vi "meta_findFirstBlock.vi"(8 "error in":errorcluster, 10 "block type":T2, 11 "meta file in":T3) -> (0 "error out":errorcluster, 1 "index":i32, 2 "block out":T1={"Version"=14, "Type"=enum."File", "Length"=0, "Data"=""}, 3 "meta file out":T3)   [LabVIEW 2017, in "NI_ExcelFile.lvlib"]
uses:
  <vilib>/express/express shared/NI_ExcelFile/NI_ExcelFile.lvlib
  <vilib>/express/express shared/NI_ExcelFile/Ctrls/meta_BlockType.ctl
  <vilib>/express/express shared/NI_ExcelFile/Ctrls/meta_file.ctl
  <vilib>/express/express shared/NI_ExcelFile/Ctrls/meta_Block.ctl
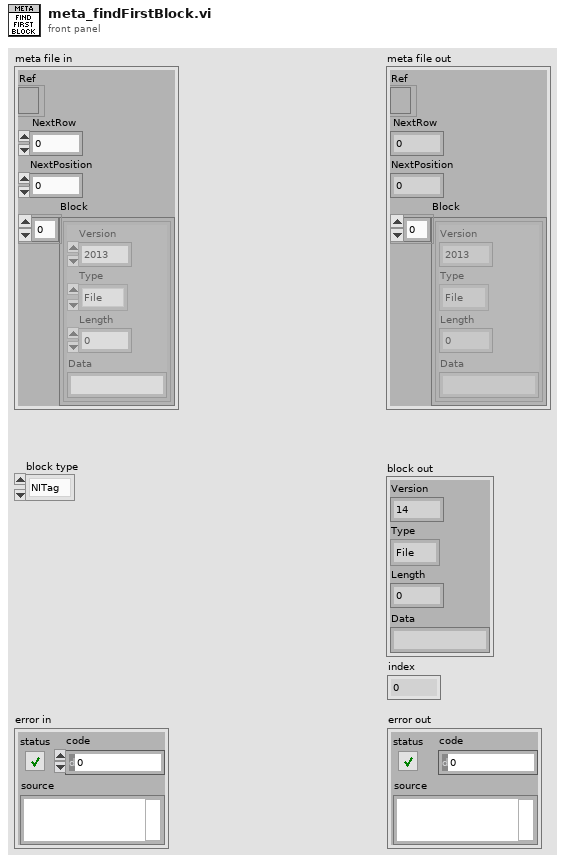
[diagram p1: front panel]
types:
  T1 = typedef "NI_ExcelFile.lvlib/meta_Block.ctl" = cluster{"Version":u16, "Type":T2, "Length":i32, "Data":string}
  T2 = typedef "NI_ExcelFile.lvlib/meta_BlockType.ctl" = enum16{"NITag", "File", "Column"}
  T3 = typedef "NI_ExcelFile.lvlib/meta_file.ctl" = cluster{"Ref":refnum<file>, "NextRow":i32, "NextPosition":i64, "Block":T1[]}
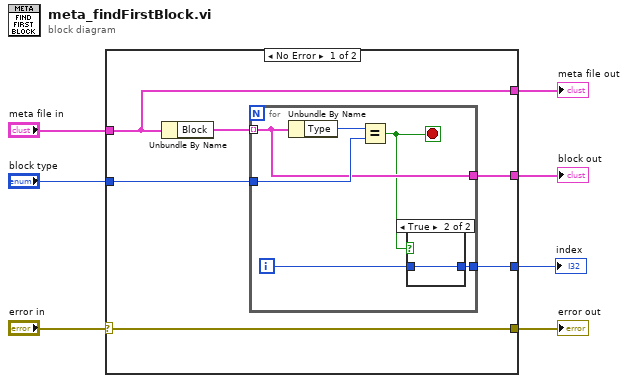
[diagram p0: block diagram]
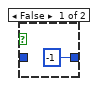
[diagram p2: hidden frame]
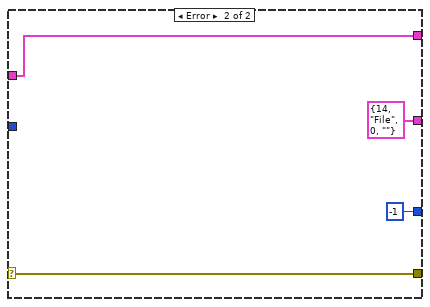
[diagram p3: hidden frame]
diagram:
  n1 = case shown="No Error" "error in" {
    selector: "error in" -> [w11 w25]
    tunnel: [w11 w25] -> w6
    tunnel: "meta file in" -> [w9 w24]
    tunnel: "block type" -> [w12 _]
    tunnel: [w10 T1 {"Version"=14, "Type"=enum."File", "Length"=0, "Data"=""} ("Block")] -> w3
    tunnel: [w9 w24] -> w2
    tunnel: [w8 -1] -> w1
    frame No Error {
      n2 = Unbundle By Name(w9) -> ("Block"=w13:T1[])
      n3 = for {
        tunnel: w13 -> [w17] mode=indexing
        tunnel: w12 -> [w18]
        tunnel: [w17] -> w10
        tunnel: [w15] -> w8
        i -> [w14]
        stop <- w16 stop-if-true
        n4 = Unbundle By Name(w17) -> ("Type"=w19:T2)
        n5 = Equal?(x=w19, y=w18) -> (x = y?=w16:bool)
        n6 = case shown="True" w16 {
          tunnel: [-1 w21] -> w15
          tunnel: w14 -> [_ w21]
          frame False {
          }
          frame True {
          }
        }
      }
    }
    frame Error {
    }
  }
  "error out" <- w6
  "meta file out" <- w2
  "block out" <- w3
  "index" <- w1
